vi "OnResize2.vi"(0 "XRef":T9, 1 "Bounds":T7, 2 "Mouse Mods":T5, 3 "State In":T1) -> (14 "Reply":T3, 15 "Fatal Error Out":T2, 16 "State Out":T1)   [LabVIEW 2015, in "Build JSON Array.xnode"]
uses:
  Build JSON Array.xnode
  <vilib>/XNodeSupport/XNodeXNodeRef.ctl
  <vilib>/XNodeSupport/XNodeRect32.ctl
  <vilib>/XNodeSupport/XNodeInt.ctl
  <vilib>/XNodeSupport/XNodeMouseMods.ctl
  <vilib>/XNodeSupport/XNodeBool.ctl
  State.ctl
  <vilib>/XNodeSupport/XNodeStringArray.ctl
  <vilib>/XNodeSupport/XNodeString.ctl
  <vilib>/XNodeSupport/XNodeErrorCluster.ctl
  dimensions.vi
  <vilib>/XNodeSupport/NI_XNodeSupport.lvlib
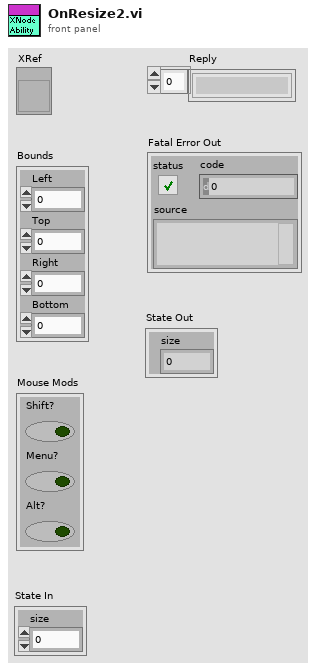
[diagram p1: front panel]
types:
  T1 = typedef "Build JSON Array.xnode/State.ctl" = cluster{"size":u32}
  T2 = typedef "NI_XNodeSupport.lvlib/XNodeErrorCluster.ctl" = errorcluster
  T3 = typedef "NI_XNodeSupport.lvlib/XNodeStringArray.ctl" = T4[]
  T4 = typedef "NI_XNodeSupport.lvlib/XNodeString.ctl" = string
  T5 = typedef "NI_XNodeSupport.lvlib/XNodeMouseMods.ctl" = cluster{"Shift?":T6, "Menu?":T6, "Alt?":T6}
  T6 = typedef "NI_XNodeSupport.lvlib/XNodeBool.ctl" = bool
  T7 = typedef "NI_XNodeSupport.lvlib/XNodeRect32.ctl" = cluster{"Left":T8, "Top":T8, "Right":T8, "Bottom":T8}
  T8 = typedef "NI_XNodeSupport.lvlib/XNodeInt.ctl" = i32
  T9 = typedef "NI_XNodeSupport.lvlib/XNodeXNodeRef.ctl" = refnum<vi>
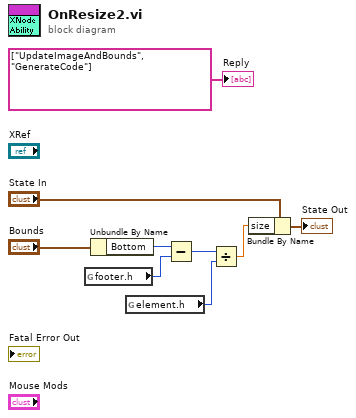
[diagram p0: block diagram]
diagram:
  n1 = global read "dimensions.vi" "footer.h"() -> (w2:i16)
  n2 = Unbundle By Name("Bounds") -> ("Bottom"=w3:T8)
  n3 = global read "dimensions.vi" "element.h"() -> (w5:i16)
  n4 = Subtract(x=w3, y=w2) -> (x-y=w1:T8)
  n5 = Divide(x=w1, y=w5) -> (x/y=w4:dbl)
  n6 = Bundle By Name(cluster="State In", "size"=w4) -> (→"State Out":T1)
  "Reply" <- T3 ["UpdateImageAndBounds", "GenerateCode"] ("Reply")
